vi "Query Mask Test Results.vi"(8 "error in (no error)":errorcluster, 11 "VISA resource name":refnum<visa-resource-name>) -> (0 "error out":errorcluster, 1 "Region Failures":dbl[](array[numeric])=[0.0, 196443.0, 228581.0], 2 "Acquired Waveforms":dbl, 3 "VISA resource name out":refnum<visa-resource-name>, 5 "Failed Waveforms":dbl, 7 "Mask Regions":i32)   [LabVIEW 2020, in "Agilent 90000 Series.lvlib"]
doc: "Returns the results of the Mask Test."
uses:
  Agilent 90000 Series.lvlib
panel:
  # "This array is zero \nindexed. Hence\nthe zero indexed value\ncorresponds to Region 1"
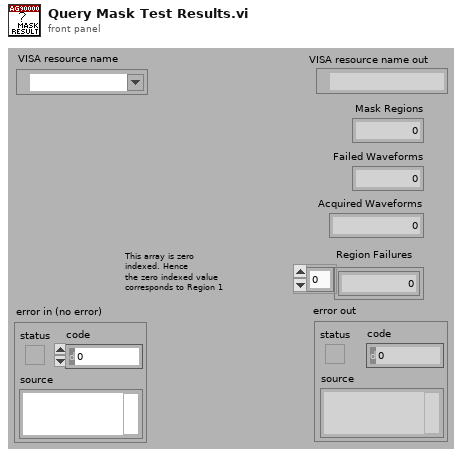
[diagram p1: front panel]
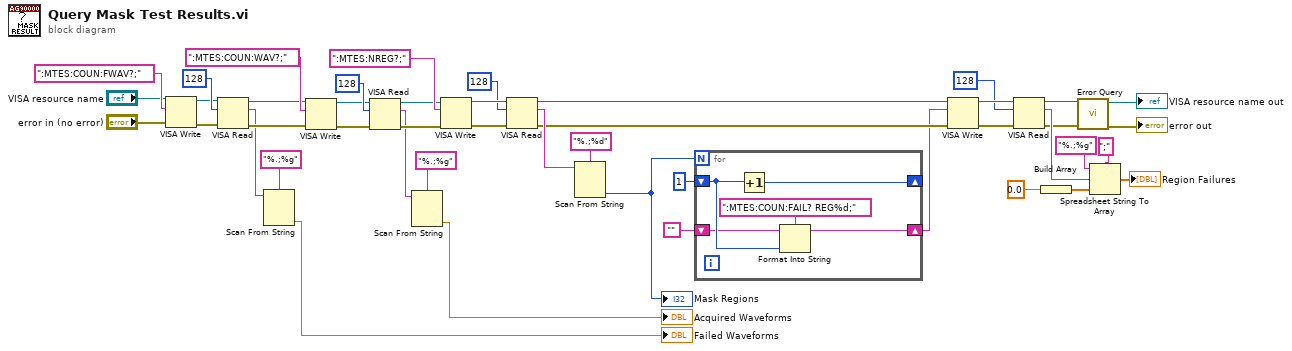
[diagram p0: block diagram]
diagram:
  n1 = VISA Write(VISA resource name="VISA resource name", write buffer=":MTES:COUN:FWAV?;", error in (no error)="error in (no error)") -> (VISA resource name out=w15:refnum<visa-resource-name>, error out=w14:errorcluster)  [unwired: 1 out]
  n2 = VISA Read(VISA resource name=w15, byte count=u32 128, error in (no error)=w14) -> (VISA resource name out=w12:refnum<visa-resource-name>, read buffer=w6:string, error out=w11:errorcluster)  [unwired: 1 out]
  n3 = Scan From String(format string="%.;%g", input string=w6) -> (output 1=→"Failed Waveforms":dbl)  [unwired: 2 in, 4 out]
  n4 = VISA Write(VISA resource name=w12, write buffer=":MTES:COUN:WAV?;", error in (no error)=w11) -> (VISA resource name out=w10:refnum<visa-resource-name>, error out=w9:errorcluster)  [unwired: 1 out]
  n5 = VISA Read(VISA resource name=w10, byte count=u32 128, error in (no error)=w9) -> (VISA resource name out=w8:refnum<visa-resource-name>, read buffer=w5:string, error out=w7:errorcluster)  [unwired: 1 out]
  n6 = Scan From String(format string="%.;%g", input string=w5) -> (output 1=→"Acquired Waveforms":dbl)  [unwired: 2 in, 4 out]
  n7 = VISA Write(VISA resource name=w8, write buffer=":MTES:NREG?;", error in (no error)=w7) -> (VISA resource name out=w45:refnum<visa-resource-name>, error out=w44:errorcluster)  [unwired: 1 out]
  n8 = VISA Read(VISA resource name=w45, byte count=u32 128, error in (no error)=w44) -> (VISA resource name out=w38:refnum<visa-resource-name>, read buffer=w43:string, error out=w37:errorcluster)  [unwired: 1 out]
  n9 = Scan From String(format string="%.;%d", input string=w43) -> (output 1=w39:i32)  [unwired: 2 in, 4 out]
  "Mask Regions" <- w39
  n10 = for {
    N: w39 -> [_]
    shift-right: [w48] -> _
    shift-left: u32 1 -> [w49]
    shift-right: [w47] -> w30
    shift-left: "" -> [w46]
    n11 = Increment(x=w49) -> (x+1=w48:u32)
    n12 = Format Into String(format string=":MTES:COUN:FAIL? REG%d;", initial string=w46, w49) -> (resulting string=w47:string)  [unwired: 1 in, 1 out]
  }
  n13 = VISA Write(VISA resource name=w38, write buffer=w30, error in (no error)=w37) -> (VISA resource name out=w36:refnum<visa-resource-name>, error out=w35:errorcluster)  [unwired: 1 out]
  n14 = VISA Read(VISA resource name=w36, byte count=u32 128, error in (no error)=w35) -> (VISA resource name out=w24:refnum<visa-resource-name>, read buffer=w31:string, error out=w23:errorcluster)  [unwired: 1 out]
  n15 = Build Array(0.0 ("element")) -> (w29:dbl[])
  n16 = call "Error Query.vi"("error in (no error)"=w23, "VISA resource name"=w24) -> ("error out"=→"error out":errorcluster, "VISA resource name out"=→"VISA resource name out":refnum<visa-resource-name>)  [unwired: 8 out]
  n17 = Spreadsheet String To Array(delimiter (Tab)=";", format string="%.;%g", spreadsheet string=w31, array type (2D Dbl)=w29) -> (array=→"Region Failures":dbl[])
